vi "ZaberTest.vi"() -> ()   [LabVIEW 2013]
uses:
  <instrlib>/ZaberTSeries/ZaberTSeries.lvlib
panel:
  in  "Go":bool
  in  "String command (Home)":string
  in  "stop":bool
  out "double precision float":dbl
  in  "VISA resource name":refnum<visa-resource-name>
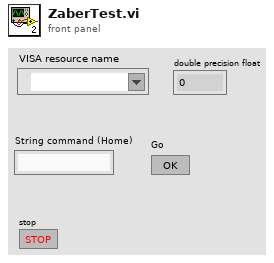
[diagram p1: front panel]
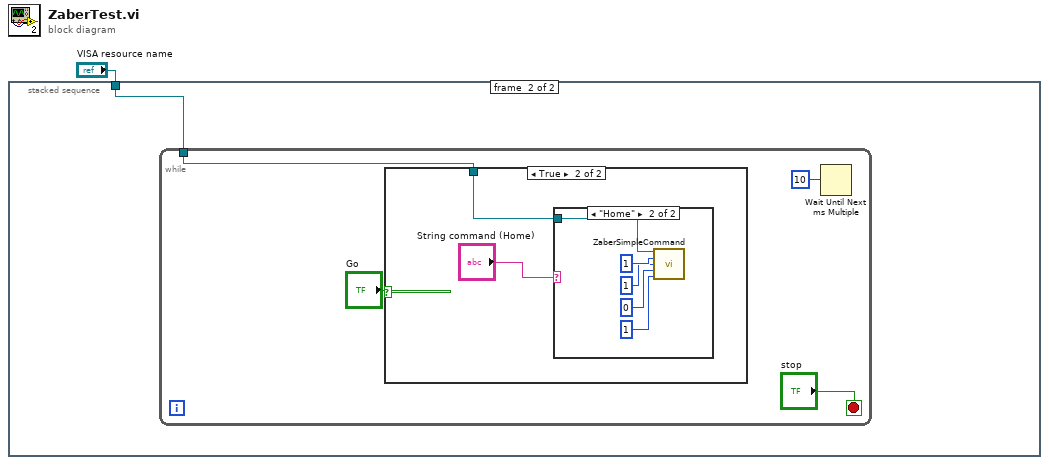
[diagram p0: block diagram]
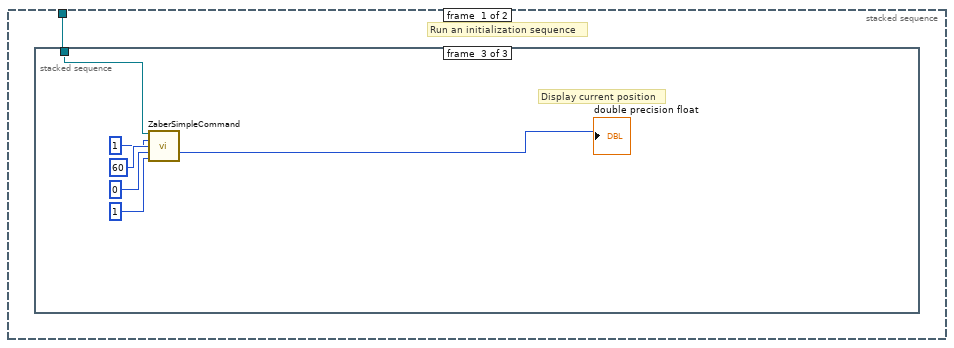
[diagram p2: hidden frame]
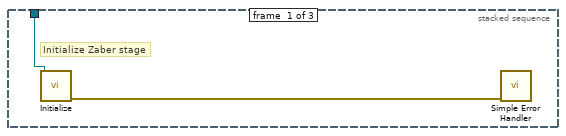
[diagram p3: hidden frame]
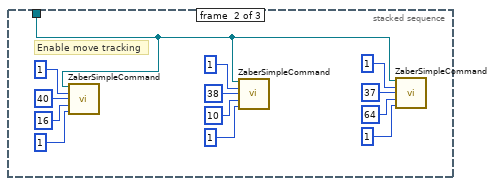
[diagram p4: hidden frame]
diagram:
  n1 = stacked-sequence {
    tunnel: "VISA resource name" -> [w2 w24]
    frame #0 {
      # "Run an initialization sequence"
      n2 = stacked-sequence {
        tunnel: w2 -> [w3 w5 w19]
        frame #0 {
          # "Initialize Zaber stage"
          n3 = call <instrlib>:"Initialize.vi"("VISA resource name"=w3) -> ("error out"=w4:errorcluster)  [unwired: 8 in, 2 out]
          n4 = call <vilib>:"Simple Error Handler.vi"("error in (no error)"=w4) -> ()  [unwired: 4 in, 5 out]
        }
        frame #1 {
          # "Enable move tracking"
          n5 = call "ZaberSimpleCommand.vi"("VISA Refnum in"=w5, "Num1"=1, "Cmd"=40, "Val"=16, "Resp num"=1) -> ()  [unwired: 8 in, 3 out]
          n6 = call "ZaberSimpleCommand.vi"("VISA Refnum in"=w5, "Num1"=1, "Cmd"=38, "Val"=10, "Resp num"=1) -> ()  [unwired: 8 in, 3 out]
          n7 = call "ZaberSimpleCommand.vi"("VISA Refnum in"=w5, "Num1"=1, "Cmd"=37, "Val"=64, "Resp num"=1) -> ()  [unwired: 8 in, 3 out]
        }
        frame #2 {
          # "Display current position"
          n8 = call "ZaberSimpleCommand.vi"("VISA Refnum in"=w19, "Num1"=1, "Cmd"=60, "Val"=0, "Resp num"=1) -> ("Val"=→"double precision float":i32)  [unwired: 8 in, 2 out]
        }
      }
    }
    frame #1 {
      n9 = while {
        tunnel: w24 -> [w26]
        stop <- "stop" stop-if-true
        n10 = case shown="True" "Go" {
          tunnel: w26 -> [_ w30]
          frame False {
          }
          frame True {
            n11 = case shown="\"Home\"" "String command (Home)" {
              tunnel: w30 -> [_ w31]
              frame "False", Default {
              }
              frame "Home" {
                n12 = call "ZaberSimpleCommand.vi"("VISA Refnum in"=w31, "Num1"=1, "Cmd"=1, "Val"=0, "Resp num"=1) -> ()  [unwired: 8 in, 3 out]
              }
            }
          }
        }
        n13 = Wait Until Next ms Multiple(millisecond multiple=10) -> ()  [unwired: 1 out]
      }
    }
  }
